vi "Change Motor ID.vi"(8 "error in (no error)":errorcluster, 9 "New ID":u8, 10 "Current ID":u8, 11 "VISA resource name":refnum<visa-resource-name>) -> (0 "error out":errorcluster, 3 "VISA Resource Out":refnum<visa-resource-name>)   [LabVIEW 2016, in "Dynamixel Motor.lvlib"]
doc: "Changes a motor's ID."
uses:
  Dynamixel Motor.lvlib
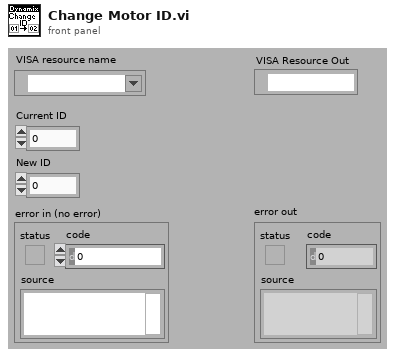
[diagram p1: front panel]
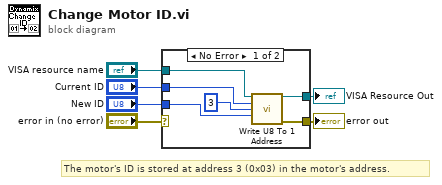
[diagram p0: block diagram]
diagram:
  # "The motor's ID is stored at address 3 (0x03) in the motor's address."
  n1 = case shown="No Error" "error in (no error)" {
    selector: "error in (no error)" -> [_ w14]
    tunnel: [w10 w14] -> w3
    tunnel: [w11 w13] -> w2
    tunnel: "VISA resource name" -> [w12 w13]
    tunnel: "Current ID" -> [w8 _]
    tunnel: "New ID" -> [w7 _]
    frame No Error {
      n2 = call "Write U8 To 1 Address.vi"("VISA resource name"=w12, "Motor ID (0)"=w8, "Address number (0)"=u8 3 ("Address"), "Parameter (0)"=w7) -> ("VISA resource name out"=w11:refnum<visa-resource-name>, "error out"=w10:errorcluster)  [unwired: 10 in]
    }
    frame Error {
    }
  }
  "error out" <- w3
  "VISA Resource Out" <- w2
